vi "2.2 OverrideHandler.vi"() -> ()   [LabVIEW 2011]
uses:
  2 Typedefs/setpoints to boat.ctl
  2 Typedefs/sail setpt.ctl
  2 Typedefs/rudder angle.ctl
  2 Globals/2 Global.vi
panel:
  out "Think Setpoints":cluster{"Rudder Angle":T1, "Sail Position":T2}
  out "Override Active":bool
  out "Override Setpoints":T3
  out "Setpoints to Boat":T3
  # "This is the Override Handler: \nIt checks to see if the manual override has been activated, and sends setpoints to the boat based on that boolean.\n\nTODO: Check to make sure that rudder and sail are always communicated as (0) = rudder and (1) = sail."
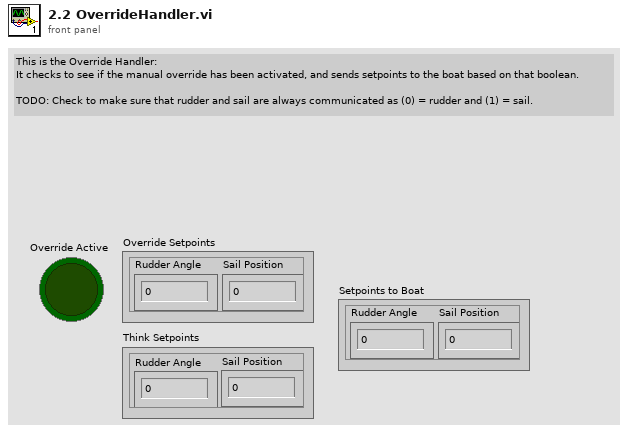
[diagram p1: front panel]
types:
  T1 = typedef "rudder angle.ctl" = dbl
  T2 = typedef "sail setpt.ctl" = dbl
  T3 = typedef "setpoints to boat.ctl" = cluster{"Sail Position":T2, "Rudder Angle":T1}
  T4 = typedef "manual override.ctl" = cluster{"Override Active":bool, "Setpoints":T3}
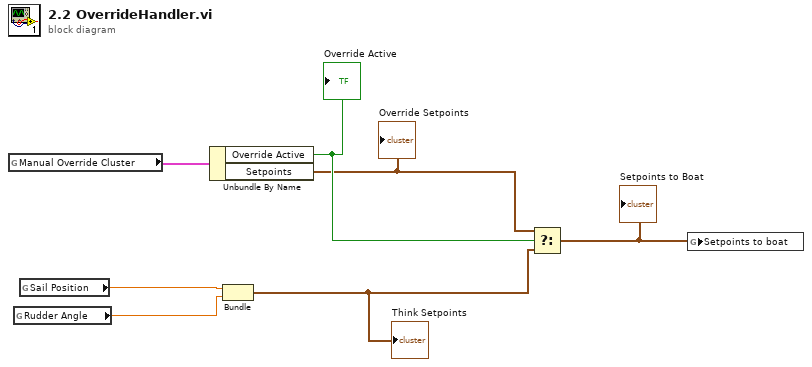
[diagram p0: block diagram]
diagram:
  n1 = global read "2 Global.vi" "Manual Override Cluster"() -> (w7:T4)
  n2 = global read "2 Global.vi" "Rudder Angle"() -> (w3:T1)
  n3 = global read "2 Global.vi" "Sail Position"() -> (w4:T2)
  n4 = Unbundle By Name(w7) -> ("Override Active"=w6:bool, "Setpoints"=w5:T3)
  "Override Setpoints" <- w5
  "Override Active" <- w6
  n5 = Bundle("Sail Position"=w4, "Rudder Angle"=w3) -> (w1:cluster{"Sail Position":T2, "Rudder Angle":T1})  [unwired: 1 in]
  "Think Setpoints" <- w1
  n6 = Select(t=w5, s=w6, f=w1) -> (s? t:f=w2:T3)
  "Setpoints to Boat" <- w2
  n7 = global write "2 Global.vi" "Setpoints to boat"(w2) -> ()
